vi "Check String Type.vi"(8 "error in (no error)":errorcluster, 10 "String":string, 11 "String Value in":refnum<class "String Value.lvclass">) -> (0 "error out":errorcluster, 3 "String Value out":refnum<class "String Value.lvclass">)   [LabVIEW 2020]
uses:
  String Value.lvclass
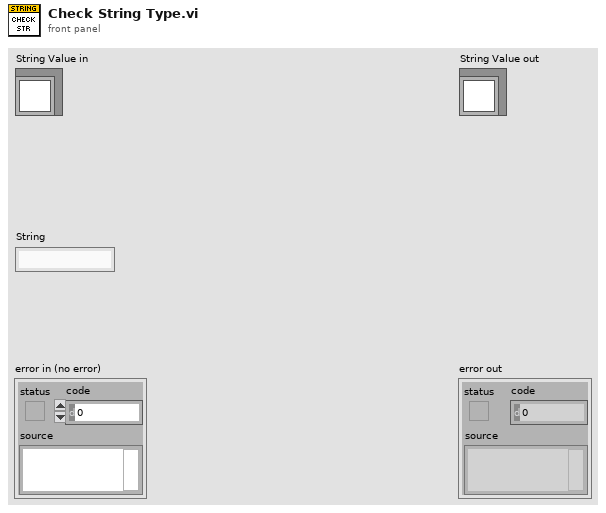
[diagram p1: front panel]
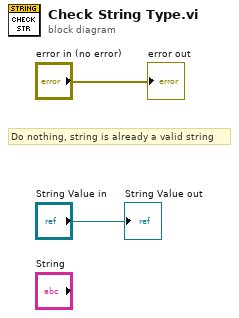
[diagram p0: block diagram]
diagram:
  # "Do nothing, string is already a valid string"
  "error out" <- "error in (no error)"
  "String Value out" <- "String Value in"
